vi "fixgraphs.vi"(6 "Scan Parameters":T1 {"fill frac" min=0.0 max=1.0 step=0.05; "y voltage max" format="%0.2p"; "y voltage min" format="%0.2p"; "x voltage max" format="%0.2p"; "x voltage min" format="%0.2p"}, 9 "IntGraph Refnum 3":refnum<vi>, 10 "IntGraph Refnum in":refnum<vi>, 11 "IntensityGraph in":refnum<vi>) -> ()   [LabVIEW 2012]
uses:
  typedefs/Scan Parameters.ctl
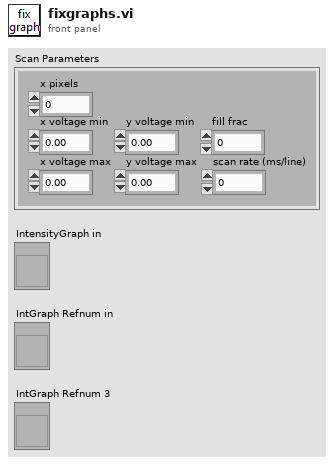
[diagram p1: front panel]
types:
  T1 = typedef "Scan Parameters.ctl" = cluster{"x pixels":i32, "x voltage min":dbl, "x voltage max":dbl, "y voltage min":dbl, "y voltage max":dbl, "fill frac":dbl, "Zoom":dbl, "BiDi":bool, "scan rate (ms/line)":dbl}
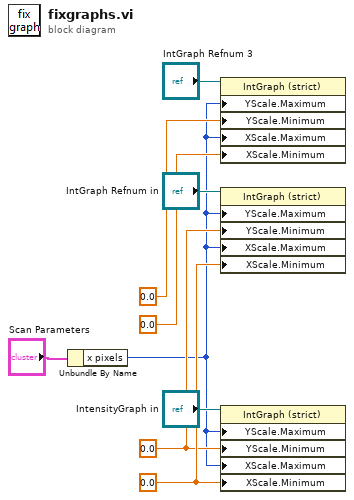
[diagram p0: block diagram]
diagram:
  w6 = 0.0 ("Y Scale.Range:Minimum")
  w5 = 0.0 ("Y Scale.Range:Minimum")
  n1 = Unbundle By Name("Scan Parameters") -> ("x pixels"=w1:i32)
  n2 = property on="Property Node" class="IntGraph (strict)"(reference="IntGraph Refnum 3", "YScale.Maximum"=w1, "YScale.Minimum"=0.0 ("Y Scale.Range:Minimum"), "XScale.Maximum"=w1, "XScale.Minimum"=0.0 ("Y Scale.Range:Minimum")) -> ()  [unwired: 1 in, 2 out]
  n3 = property on="Property Node" class="IntGraph (strict)"(reference="IntGraph Refnum in", "YScale.Maximum"=w1, "YScale.Minimum"=w5, "XScale.Maximum"=w1, "XScale.Minimum"=w6) -> ()  [unwired: 1 in, 2 out]
  n4 = property on="Property Node" class="IntGraph (strict)"(reference="IntensityGraph in", "YScale.Maximum"=w1, "YScale.Minimum"=w5, "XScale.Maximum"=w1, "XScale.Minimum"=w6) -> ()  [unwired: 1 in, 2 out]
